vi "Save-Load Initial Values.vi"(6 "Which file? (User profile.ini)":T1=enum."Loaded User profile.ini", 8 "error in":errorcluster, 11 "Function":T2=enum."Load from file") -> (0 "error out":errorcluster)   [LabVIEW 2013]
uses:
  Typedefs/Save-Load enum.ctl
  Typedefs/Which path.ctl
  User Interface/User profiles code/Typedefs/Comparison states.ctl
  <vilib>/Utility/config.llb/NI_LVConfig.lvlib
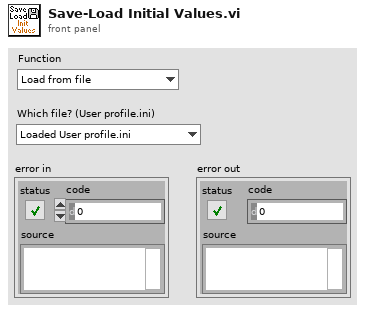
[diagram p1: front panel]
types:
  T1 = typedef "Which path.ctl" = enum16{"Configuration Files", "Calibration Files", "Images", "Setup.ini", "Loaded User profile.ini", "User's-Previous session.ini", "New user profile.ini", "Selected User profile.ini", "User profiles folder", "Power meter scaling.txt", "FOV Cal.ini"}
  T2 = typedef "Save-Load enum.ctl" = enum16{"Save to file", "Load from file", "Compare from file"}
  T3 = typedef "Ini file interface (DBL).ctl" = cluster{"key":string, "Save?":bool, "Default":dbl}[]
  T4 = typedef "NI_LVConfig.lvlib/Config Data RefNum.ctl" = refnum<k1>
  T5 = typedef "Ini file interface (String).ctl" = cluster{"key":string, "Save?":bool, "Default":string}[]
  T6 = typedef "Ini file interface (Boolean).ctl" = cluster{"key":string, "Save?":bool, "Default":bool}[]
  T7 = typedef "Comparison states.ctl" = enum16{"Init.", "Add", "Read"}
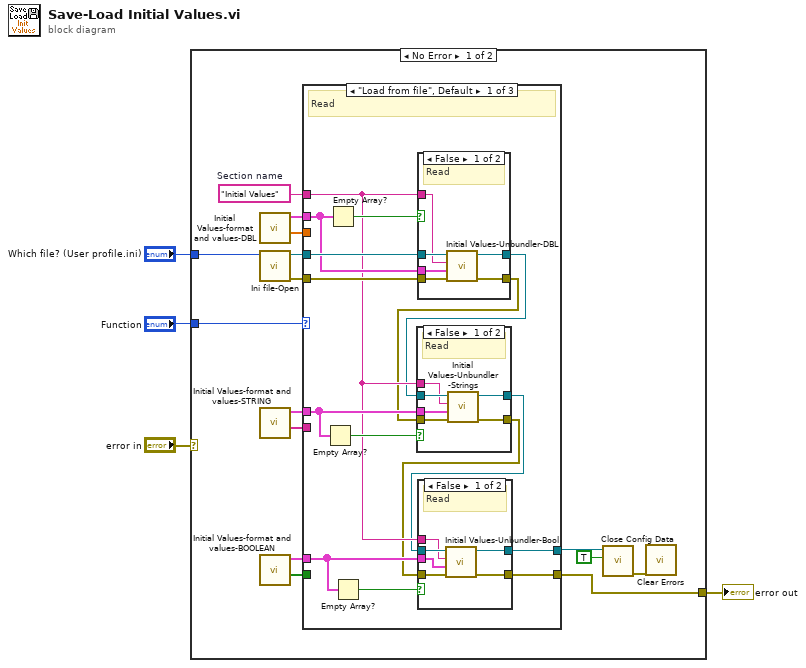
[diagram p0: block diagram]
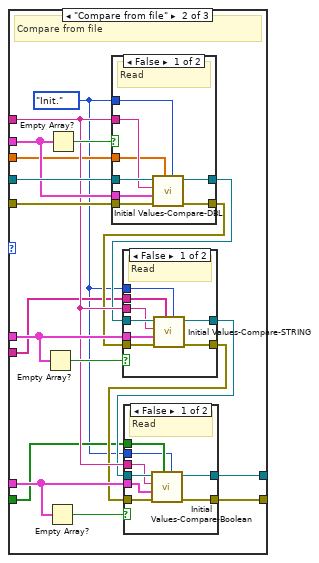
[diagram p5: hidden frame]
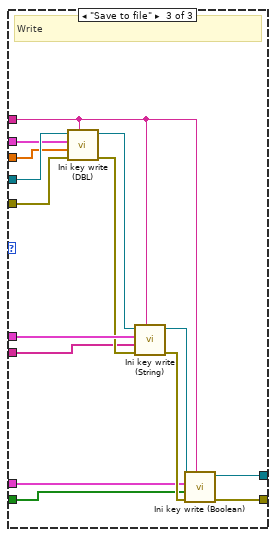
[diagram p9: hidden frame]
diagram:
  n1 = case shown="No Error" "error in" {
    selector: "error in" -> [_ w123]
    tunnel: [w13 w123] -> w4
    tunnel: "Which file? (User profile.ini)" -> [w6 _]
    tunnel: "Function" -> [w5 _]
    frame No Error {
      w19 = "Initial Values"  # Section name
      n2 = call "Initial Values-format and values-DBL.vi"() -> ("Values Array"=w11:dbl[], "Keys Array"=w12:T3)  [unwired: 10 in]
      n3 = call "Ini file-Open.vi"("Which file?"=w6) -> ("error out"=w16:errorcluster, "User profile ini file ref"=w17:T4)  [unwired: 7 in, 2 out]
      n4 = call "Initial Values-format and values-STRING.vi"() -> ("Values Array"=w9:string[], "Keys Array"=w10:T5)  [unwired: 10 in]
      n5 = call "Initial Values-format and values-BOOLEAN.vi"() -> ("Values Array"=w7:bool[], "Keys Array"=w8:T6)  [unwired: 10 in]
      n6 = case shown="\"Load from file\", Default" w5 {
        tunnel: [w29 w72 w109] -> w13
        tunnel: [w30 w73 w108] -> w15
        tunnel: w16 -> [w31 w74 w121]
        tunnel: w17 -> [w34 w77 w122]
        tunnel: w19 -> [w24 w67 w111]
        tunnel: w12 -> [w33 w76 w119]
        tunnel: w11 -> [_ w62 w120]
        tunnel: w7 -> [_ w61 w110]
        tunnel: w8 -> [w28 w71 w112]
        tunnel: w9 -> [_ w60 w115]
        tunnel: w10 -> [w25 w68 w118]
        frame "Load from file", Default {
          # "Read"
          n7 = Empty Array?(array=w25) -> (empty?=w26:bool)
          n8 = Empty Array?(array=w33) -> (empty?=w32:bool)
          n9 = Empty Array?(array=w28) -> (empty?=w27:bool)
          n10 = case shown="False" w32 {
            tunnel: w34 -> [w56 w58]
            tunnel: [w55 w58] -> w20
            tunnel: [w54 w57] -> w21
            tunnel: w31 -> [w53 w57]
            tunnel: w24 -> [w51 _]
            tunnel: w33 -> [w52 _]
            frame False {
              # "Read"
              n11 = call "Initial Values-Unbundler-DBL.vi"("error in (no error)"=w53, "Keys Array"=w52, "Section name"=w51, "User profile ini file ref"=w56) -> ("error out"=w54:errorcluster, "User profile ini file ref"=w55:T4)  [unwired: 6 in]
            }
            frame True {
              # "No parametersof such type"
            }
          }
          n12 = case shown="False" w26 {
            tunnel: [w37 w42] -> w23
            tunnel: [w36 w41] -> w22
            tunnel: w25 -> [w39 _]
            tunnel: w20 -> [w40 w42]
            tunnel: w21 -> [w35 w41]
            tunnel: w24 -> [w38 _]
            frame False {
              # "Read"
              n13 = call "Initial Values-Unbundler-Strings.vi"("error in (no error)"=w35, "Keys Array"=w39, "Section name"=w38, "User profile ini file ref"=w40) -> ("error out"=w36:errorcluster, "User profile ini file ref"=w37:T4)  [unwired: 6 in]
            }
            frame True {
              # "No parametersof such type"
            }
          }
          n14 = case shown="False" w27 {
            tunnel: [w47 w50] -> w30
            tunnel: [w46 w49] -> w29
            tunnel: w28 -> [w43 _]
            tunnel: w23 -> [w48 w50]
            tunnel: w22 -> [w45 w49]
            tunnel: w24 -> [w44 _]
            frame False {
              # "Read"
              n15 = call "Initial Values-Unbundler-Bool.vi"("error in (no error)"=w45, "Keys Array"=w43, "Section name"=w44, "User profile ini file ref"=w48) -> ("error out"=w46:errorcluster, "User profile ini file ref"=w47:T4)  [unwired: 6 in]
            }
            frame True {
              # "No parametersof such type"
            }
          }
        }
        frame "Compare from file" {
          w59 = Comparison_states."Init." ("Function")
          # "Compare from file"
          n16 = Empty Array?(array=w68) -> (empty?=w69:bool)
          n17 = Empty Array?(array=w71) -> (empty?=w70:bool)
          n18 = Empty Array?(array=w76) -> (empty?=w75:bool)
          n19 = case shown="False" w75 {
            tunnel: w77 -> [w105 w107]
            tunnel: [w104 w107] -> w63
            tunnel: [w103 w106] -> w64
            tunnel: w74 -> [w102 w106]
            tunnel: w67 -> [w100 _]
            tunnel: w76 -> [w101 _]
            tunnel: w62 -> [w99 _]
            tunnel: w59 -> [w98 _]
            frame False {
              # "Read"
              n20 = call "Initial Values-Compare-DBL.vi"("Function (Add)"=w98, "Current values"=w99, "error in (no error)"=w102, "Keys Array"=w101, "Section name"=w100, "User profile ini file ref"=w105) -> ("error out"=w103:errorcluster, "User profile ini file ref"=w104:T4)  [unwired: 1 in, 3 out]
            }
            frame True {
              # "No parametersof such type"
            }
          }
          n21 = case shown="False" w69 {
            tunnel: [w82 w87] -> w66
            tunnel: [w81 w86] -> w65
            tunnel: w68 -> [w84 _]
            tunnel: w63 -> [w85 w87]
            tunnel: w64 -> [w80 w86]
            tunnel: w67 -> [w83 _]
            tunnel: w59 -> [w79 _]
            tunnel: w60 -> [w78 _]
            frame False {
              # "Read"
              n22 = call "Initial Values-Compare-STRING.vi"("Function (Add)"=w79, "Current values"=w78, "error in (no error)"=w80, "Keys Array"=w84, "Section name"=w83, "User profile ini file ref"=w85) -> ("error out"=w81:errorcluster, "User profile ini file ref"=w82:T4)  [unwired: 1 in, 3 out]
            }
            frame True {
              # "No parametersof such type"
            }
          }
          n23 = case shown="False" w70 {
            tunnel: [w94 w97] -> w73
            tunnel: [w93 w96] -> w72
            tunnel: w71 -> [w90 _]
            tunnel: w66 -> [w95 w97]
            tunnel: w65 -> [w92 w96]
            tunnel: w67 -> [w91 _]
            tunnel: w61 -> [w89 _]
            tunnel: w59 -> [w88 _]
            frame False {
              # "Read"
              n24 = call "Initial Values-Compare-Boolean.vi"("Function (Add)"=w88, "Current values"=w89, "error in (no error)"=w92, "Keys Array"=w90, "Section name"=w91, "User profile ini file ref"=w95) -> ("error out"=w93:errorcluster, "User profile ini file ref"=w94:T4)  [unwired: 1 in, 3 out]
            }
            frame True {
              # "No parametersof such type"
            }
          }
        }
        frame "Save to file" {
          # "Write"
          n25 = call "Ini key write (DBL).vi"("Section"=w111, "error in (no error)"=w121, "Values (DBL)"=w120, "Ini file interface"=w119, "Ini file refnum in"=w122) -> ("error out"=w116:errorcluster, "Ini file refnum out"=w117:T4)  [unwired: 5 in]
          n26 = call "Ini key write (String).vi"("Section"=w111, "error in (no error)"=w116, "Values (String)"=w115, "Ini file interface"=w118, "Ini file refnum in"=w117) -> ("error out"=w113:errorcluster, "Ini file refnum out"=w114:T4)  [unwired: 5 in]
          n27 = call "Ini key write (Boolean).vi"("Section"=w111, "error in (no error)"=w113, "Values (Boolean)"=w110, "Ini file interface"=w112, "Ini file refnum in"=w114) -> ("error out"=w109:errorcluster, "Ini file refnum out"=w108:T4)  [unwired: 5 in]
        }
      }
      n28 = call <vilib>:"Close Config Data.vi"("write file if changed (T)"=TRUE ("write configuration file? (F)"), "refnum"=w15) -> ("error out"=w14:errorcluster)  [unwired: 8 in, 1 out]
      n29 = call <vilib>:"Clear Errors.vi"("error in (no error)"=w14) -> ()  [unwired: 6 in, 1 out]
    }
    frame Error {
    }
  }
  "error out" <- w4
